vi "Create channel error check(subVI).vi"(8 "error in (no error)":errorcluster, 10 "Phisical channels":T1[](array[typedef]) items=["None", "AO1", "AO2", "AO3", "AO4", "AO5", "AO6", "AO7", "AO8", "AO9", "AO10", "AO11", "AO12", "AO13", "AO14", "AO15", "AO16"], 11 "Ranges":T2[](array[typedef])) -> (0 "error out":errorcluster)   [LabVIEW 2009, in "MicroDAQ.lvlib" / "Analog output.lvclass"]
uses:
  <instrlib>/MicroDAQ/Channel/Analog Output/Analog output.lvclass
  <instrlib>/MicroDAQ/Tools/Analo Range Enum.ctl
  <instrlib>/MicroDAQ/Tools/Analog Channel Enum.ctl
  <instrlib>/MicroDAQ/MicroDAQ.lvlib
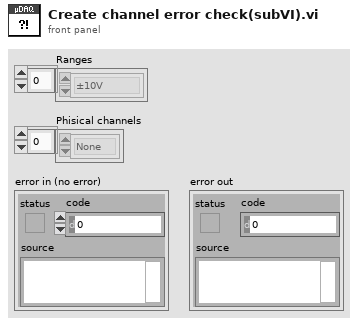
[diagram p1: front panel]
types:
  T1 = typedef "MicroDAQ.lvlib/Analog Channel Enum.ctl" = u16
  T2 = typedef "MicroDAQ.lvlib/Analo Range Enum.ctl" = enum16{"±10V", "0-10V", "±5V", "0-5V", "±5.12V", "±2.56V", "±2.5V", "±2V", "±1.24V", "±0.64V"}
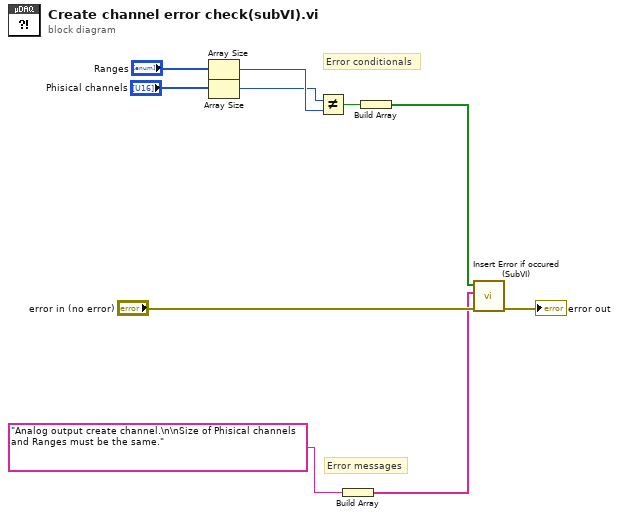
[diagram p0: block diagram]
diagram:
  # "Error messages"
  # "Error conditionals"
  n1 = Array Size(array="Ranges") -> (size(s)=w7:i32)
  n2 = Array Size(array="Phisical channels") -> (size(s)=w6:i32)
  n3 = Not Equal?(x=w6, y=w7) -> (x != y?=w5:bool)
  n4 = Build Array("Analog output create channel.\n\nSize of Phisical channels and Ranges must be the same.") -> (w2:string[])
  n5 = Build Array(w5) -> (w3:bool[])
  n6 = call <instrlib>:"Insert Error if occured (SubVI).vi"("error in (no error)"="error in (no error)", "Error messages"=w2, "Error conditionals"=w3) -> ("error out"=→"error out":errorcluster)  [unwired: 8 in]
